vi "set_all_output_names.vi"(8 "error in (no error)":errorcluster, 10 "All ouput names":string[](array[string]), 11 "VISA resource name":refnum<visa-resource-name>) -> (0 "error out":errorcluster, 3 "VISA resource name out":refnum<visa-resource-name>)   [LabVIEW 2018]
doc: "Update all output names."
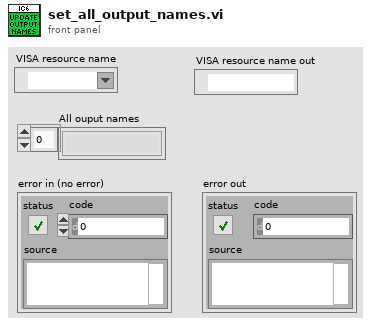
[diagram p1: front panel]
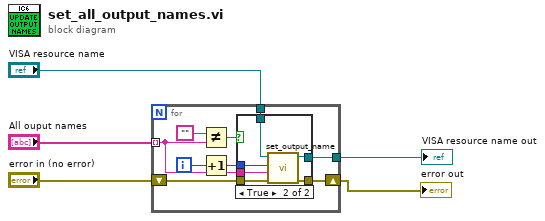
[diagram p0: block diagram]
diagram:
  n1 = for {
    tunnel: "All ouput names" -> [w10] mode=indexing
    tunnel: "VISA resource name" -> [w9]
    tunnel: [w8] -> w1
    shift-right: [w6] -> w5
    shift-left: "error in (no error)" -> [w7]
    i -> [w14]
    n2 = Not Equal?(x="", y=w10) -> (x != y?=w12:bool)
    n3 = Increment(x=w14) -> (x+1=w13:i32)
    n4 = case shown="True" w12 {
      tunnel: w13 -> [_ w21]
      tunnel: w10 -> [_ w20]
      tunnel: w9 -> [w16 w22]
      tunnel: [w16 w19] -> w8
      tunnel: [w15 w18] -> w6
      tunnel: w7 -> [w15 w17]
      frame False {
      }
      frame True {
        n5 = call "set_output_name.vi"("error in (no error)"=w17, "output name"=w20, "output number"=w21, "VISA resource name"=w22) -> ("error out"=w18:errorcluster, "VISA resource name out"=w19:refnum<visa-resource-name>)  [unwired: 6 in]
      }
    }
  }
  "error out" <- w5
  "VISA resource name out" <- w1
